vi "GEA3 Set Mix Valve Position Example.vi"() -> ()   [LabVIEW 2020]
uses:
  type defs/Data Type.ctl
  library/GEA2_Toolkit.lvlib
  type defs/ERD Write Data In.ctl
panel:
  out "Valve Offset":i16
  out "Previous Mix Valve Position":u16
  in  "MIX VALVE POSITION":i16
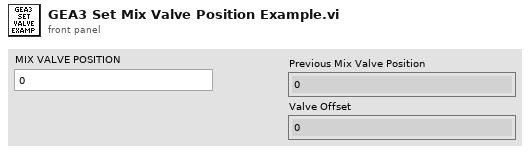
[diagram p1: front panel]
types:
  T1 = typedef "GEA2_Toolkit.lvlib/ERD Write Data In.ctl" = cluster{"ERD Number":u16, "Data Type":T2, "Data":string}
  T2 = typedef "GEA2_Toolkit.lvlib/Data Type.ctl" = enum16{"string", "boolean", "uint8_t", "uint16_t", "uint32_t", "uint64_t", "int8_t", "int16_t", "int32_t", "int64_t"}
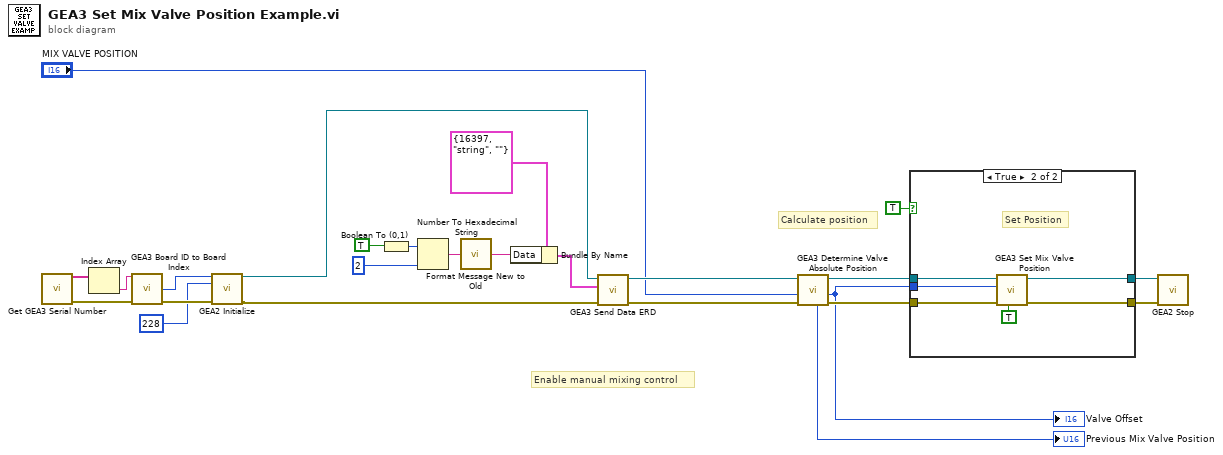
[diagram p0: block diagram]
diagram:
  # "Calculate position"
  # "Enable manual mixing control"
  n1 = call "Get GEA3 Serial Number.vi"() -> ("GEA3 Serial Numbers"=w14:string[], "Error Out"=w15:errorcluster)  [unwired: 14 in]
  n2 = Index Array(array=w14) -> (element=w13:string)  [unwired: 1 in]
  n3 = call "GEA3 Board ID to Board Index.vi"("GEA3 Serial Number"=w13, "Error In"=w15) -> ("Board Index"=w16:i32, "Error Out"=w17:errorcluster)  [unwired: 9 in, 3 out]
  n4 = call "GEA2 Initialize.vi"("Board Index"=w16, "Source Address"=u8 228, "error in"=w17) -> ("GEA2 Reference Out"=w10:refnum<k24>, "error out"=w11:errorcluster)  [unwired: 10 in, 1 out]
  n5 = Boolean To (0,1)(Boolean=TRUE) -> (0, 1=w18:i16)
  n6 = Number To Hexadecimal String(1:i16 2 ("width (-)"), 2:w18) -> (0:w20:string)
  n7 = call "Format Message New to Old.vi"("Raw Message In"=w20) -> ("Conv Message Out"=w19:string)  [unwired: 14 in]
  n8 = Bundle By Name(cluster=T1 {"ERD Number"=16397, "Data Type"=enum."string", "Data"=""} ("ERD Write Data In"), "Data"=w19) -> (w23:T1)
  n9 = call "GEA3 Send Data ERD.vi"("error in (no error)"=w11, "ERD Write Data In"=w23, ".NET Refnum in"=w10) -> ("error out"=w25:errorcluster, "GEA2 Reference Out"=w24:refnum<k24>)  [unwired: 5 in, 2 out]
  n10 = call "GEA3 Determine Valve Absolute Position.vi"("error in (no error)"=w25, "Target Position"="MIX VALVE POSITION", ".NET Refnum in"=w24) -> ("error out"=w6:errorcluster, "Valve Offset"=w5:i16, ".NET Refnum out"=w7:refnum<k24>, "Previous Mix Valve Position"=→"Previous Mix Valve Position":u16)  [unwired: 5 in]
  "Valve Offset" <- w5
  n11 = case shown="True" TRUE {
    tunnel: w7 -> [w27 w32]
    tunnel: w6 -> [w26 w31]
    tunnel: w5 -> [_ w30]
    tunnel: [w27 w29] -> w2
    tunnel: [w26 w28] -> w1
    frame False {
    }
    frame True {
      # "Set Position"
      n12 = call "GEA3 Set Mix Valve Position.vi"("Disable Check"=TRUE, "error in (no error)"=w31, "MIX VALVE STEP OFFSET (0x400A)"=w30, ".NET Refnum in"=w32) -> ("error out"=w28:errorcluster, ".NET Refnum out"=w29:refnum<k24>)  [unwired: 2 in, 4 out]
    }
  }
  n13 = call "GEA2 Stop.vi"("GEA2 Reference In"=w2, "Error In"=w1) -> ()  [unwired: 13 in, 1 out]
